vi "Area.vi"(8 "error in (no error)":errorcluster, 11 "Point in":refnum<class "PointSpecialized.lvclass">) -> (0 "error out":errorcluster, 2 "Area":T1, 3 "Point out":refnum<class "PointSpecialized.lvclass">)   [LabVIEW 2021, in "Picture2D.lvlib" / "PointSpecialized.lvclass"]
uses:
  PointSpecialized.lvclass
  PointSpecialized.lvclass/PointSpecialized.ctl
  Pen/Pen.lvclass
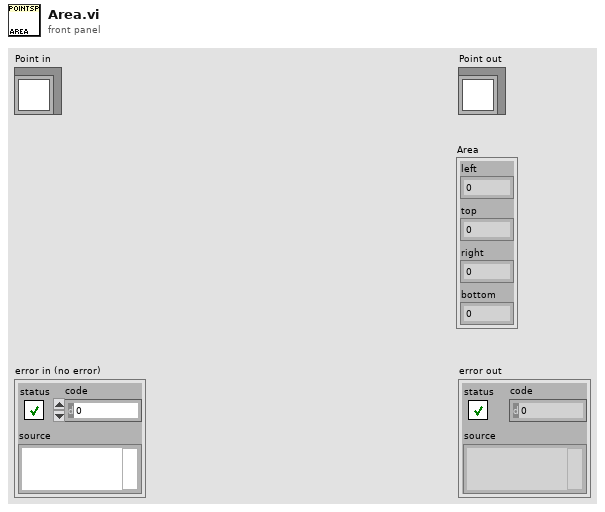
[diagram p1: front panel]
types:
  T1 = cluster{"left":i16, "top":i16, "right":i16, "bottom":i16}
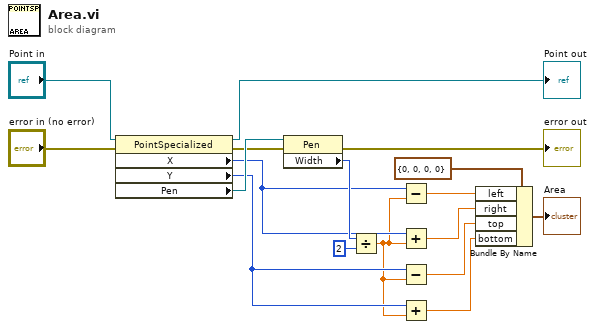
[diagram p0: block diagram]
diagram:
  n1 = property class="PointSpecialized"(reference="Point in", error in="error in (no error)") -> (reference out=→"Point out":refnum<class "PointSpecialized.lvclass">, error out=w3:errorcluster, "X"=w10:i16, "Y"=w8:i16, "Pen"=w17:refnum<class "Pen.lvclass">)
  n2 = property class="Pen"(reference=w17, error in=w3) -> (error out=→"error out":errorcluster, "Width"=w16:u16)  [unwired: 1 out]
  n3 = Divide(x=w16, y=u16 2) -> (x/y=w7:dbl)
  n4 = Subtract(x=w10, y=w7) -> (x-y=w12:dbl)
  n5 = Add(x=w10, y=w7) -> (x+y=w11:dbl)
  n6 = Subtract(x=w8, y=w7) -> (x-y=w6:dbl)
  n7 = Add(x=w8, y=w7) -> (x+y=w9:dbl)
  n8 = Bundle By Name(cluster=T1 {"left"=0, "top"=0, "right"=0, "bottom"=0} ("Area"), "left"=w12, "right"=w11, "top"=w6, "bottom"=w9) -> (→"Area":T1)
